vi "FormatowanieStringa.vi"() -> ()   [LabVIEW 2024]
uses:
  <vilib>/numeric/Random Number (Range) DBL.vi
panel:
  out "b":dbl
  out "Po彻czony String":string
  in  "a":dbl
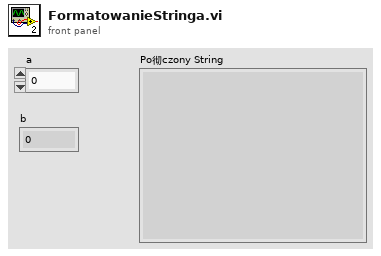
[diagram p1: front panel]
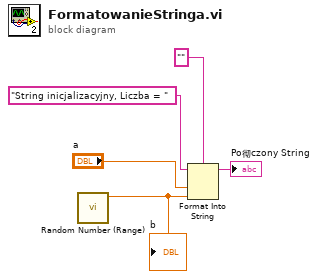
[diagram p0: block diagram]
diagram:
  n1 = call-poly <vilib>:"Random Number (Range).vi"() -> ("number"=w4:dbl)  [unwired: 11 in]
  "b" <- w4
  n2 = Format Into String(format string="", initial string="String inicjalizacyjny, Liczba = ", "a", w4) -> (resulting string=→"Po彻czony String":string)  [unwired: 1 in, 1 out]
